vi "Main.vi"(8 "error in":errorcluster, 11 "gRPC Client in":refnum<class "gRPC Client.lvclass">) -> (0 "error out":errorcluster, 3 "gRPC Client out":refnum<class "gRPC Client.lvclass">)   [LabVIEW 2023, in "gRPC Client.lvclass"]
doc: "The <b>Queued Message Handler</b> of the Worker that owns this VI."
uses:
  gRPC Client.lvclass
  C:/Program Files (x86)/National Instruments/LabVIEW 2023/vi.lib/addons/_Workers/Library/Classes/Worker/Worker.lvclass
  Generated_client/RPC Messages/streamai_signalConfig.ctl
  Generated_client/RPC Messages/streamai_SignalType.ctl
  Generated_client/RPC Messages/streamai_samplingConfig.ctl
  Initialization Data.ctl
  Response Cases.ctl
  <vilib>/gRPC/LabVIEW gRPC Library/Shared/grpcId.ctl
  gRPC Client.lvclass/gRPC Client.ctl
  <vilib>/addons/_Workers/Library/Classes/Message Queue/Message Queue.lvclass
  Generated_client/Generated_client.lvlib
  <vilib>/gRPC/LabVIEW gRPC Library/grpc-lvsupport-release.lvlib
panel:
  in  "Start Acq":bool
  in  "Address":string="localhost:50051"
  in  "Start Button":bool
  in  "Sampling Config":T1={"sample_rate"=100.0, "num_sample"=100}
  in  "Signal Config":T2={"type"=enum."SIGNAL_SQUARE", "offset"=0.0, "frequency"=5.0, "amplitude"=2.0}
  out "Waveform Chart":waveform(dbl)(graph)
  # "gRPC Client"
  # "Connector Pane"
  # "Locals"
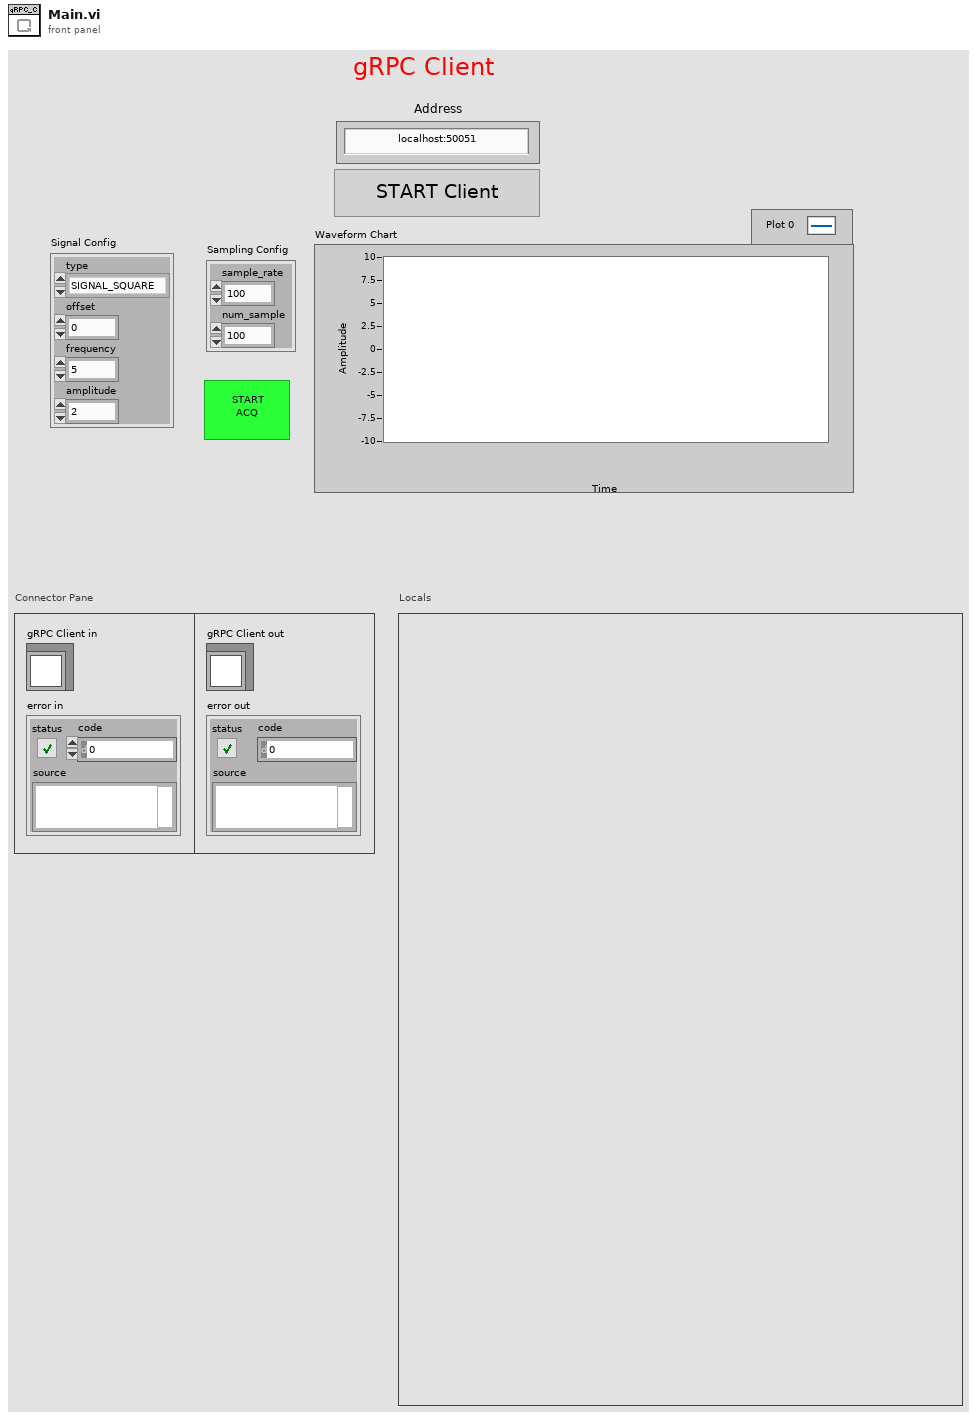
[diagram p1: front panel]
types:
  T1 = typedef "Generated_client.lvlib/streamai_samplingConfig.ctl" = cluster{"sample_rate":dbl, "num_sample":i32}
  T2 = typedef "Generated_client.lvlib/streamai_signalConfig.ctl" = cluster{"type":T3, "offset":dbl, "frequency":dbl, "amplitude":dbl}
  T3 = typedef "Generated_client.lvlib/streamai_SignalType.ctl" = enum32{"SIGNAL_SINE", "SIGNAL_SQUARE"}
  T4 = enum32{"Invalid", "Standard", "Closed", "Hidden", "Minimized", "Maximized"}
  T5 = typedef "gRPC Client.lvclass/Initialization Data.ctl" = cluster{"Response Cases":T6}
  T6 = typedef "gRPC Client.lvclass/Response Cases.ctl" = cluster{"gRPC ID":T7, "Call Id":T7}
  T7 = typedef "grpc-lvsupport-release.lvlib/grpcId.ctl" = u64
  T8 = enum8{"Enabled", "Disabled", "Disabled and Grayed Out"}
  T9 = typedef "Generated_client.lvlib/streamai_waveform.ctl" = cluster{"t0":T10, "delta_t":dbl, "values":dbl[]}
  T10 = typedef "Generated_client.lvlib/google_protobuf_Timestamp.ctl" = cluster{"seconds":i64, "nanos":i32}
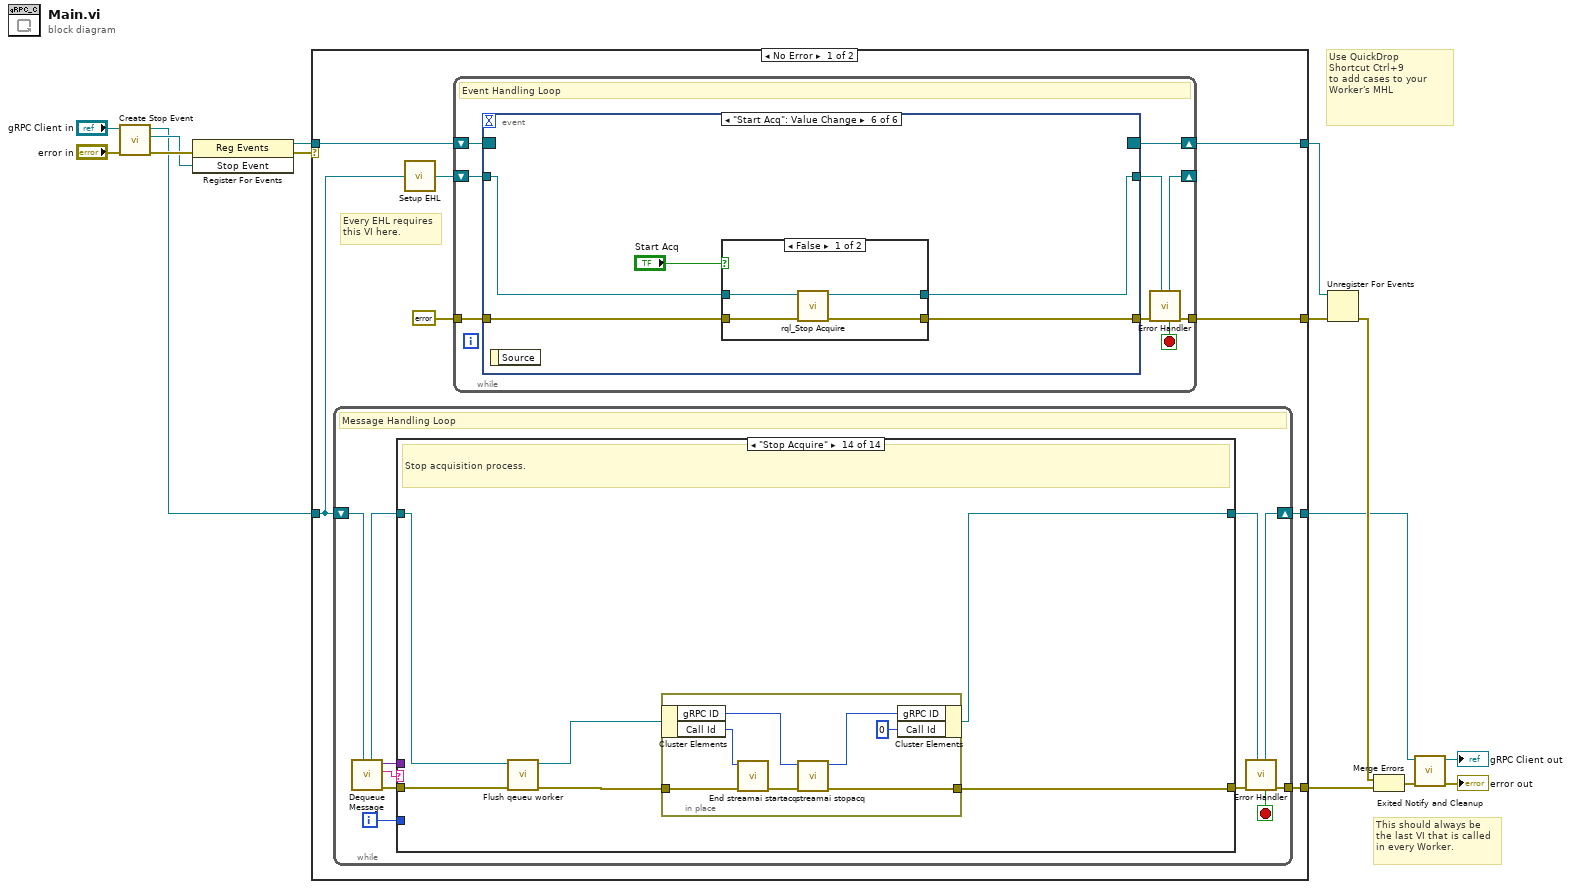
[diagram p0: block diagram]
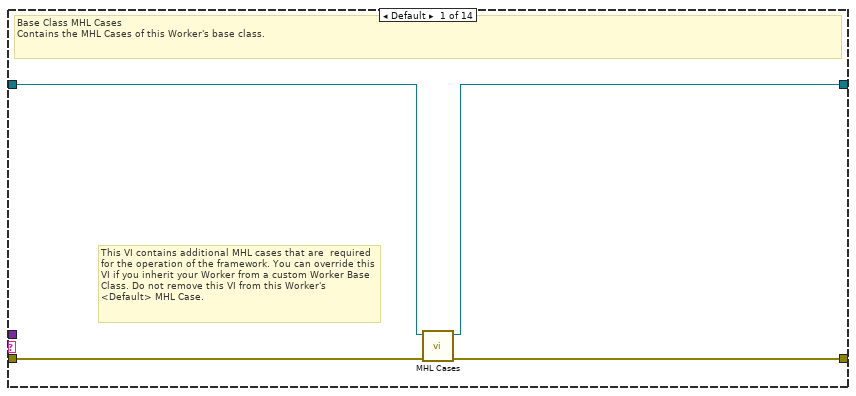
[diagram p2: hidden frame]
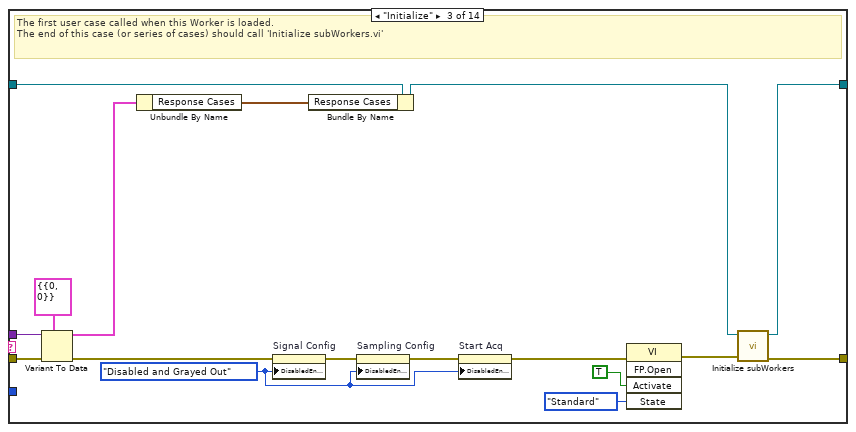
[diagram p4: hidden frame]
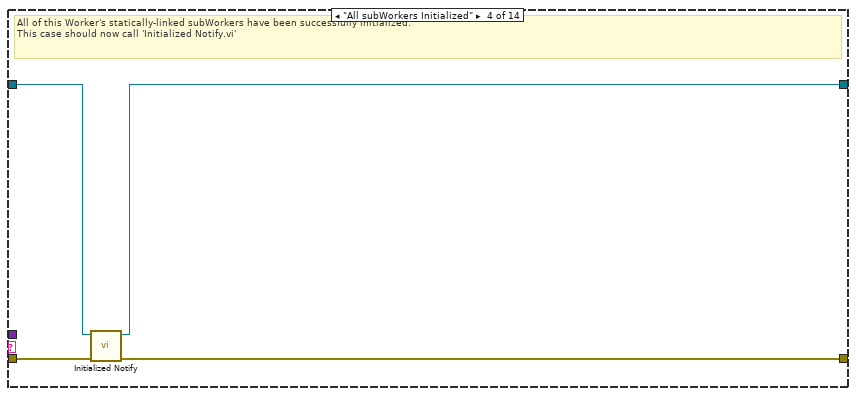
[diagram p5: hidden frame]
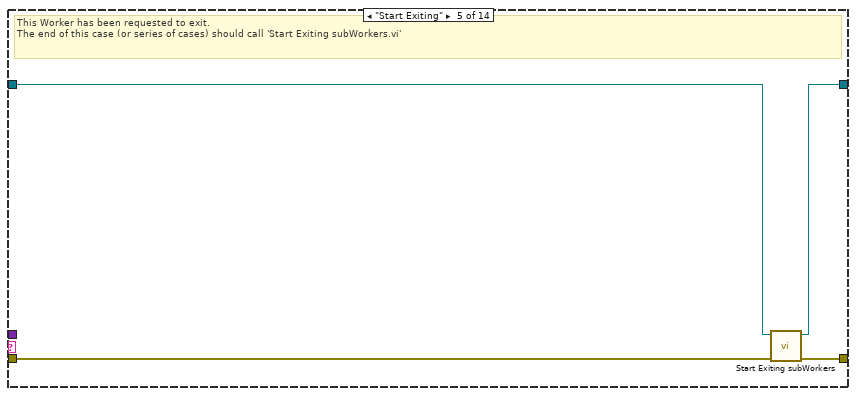
[diagram p6: hidden frame]
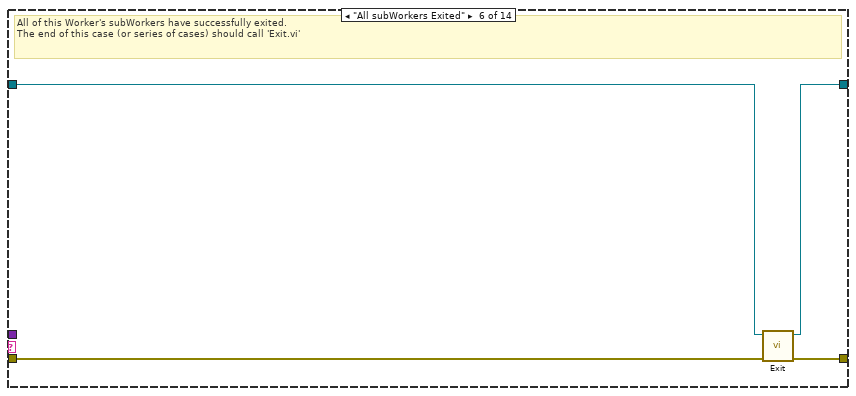
[diagram p7: hidden frame]
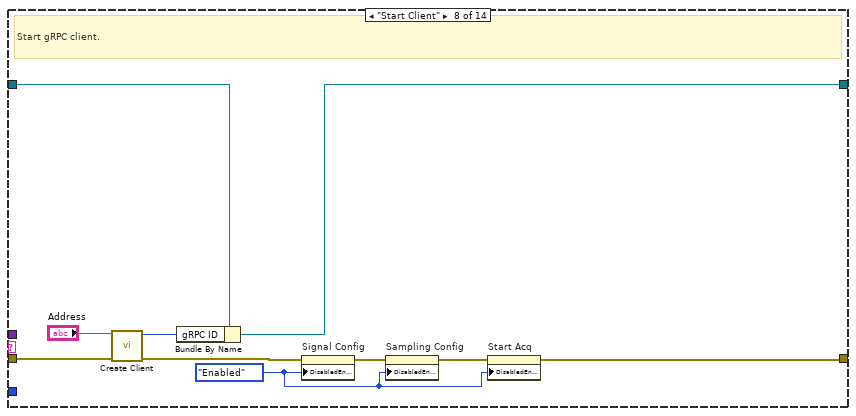
[diagram p9: hidden frame]
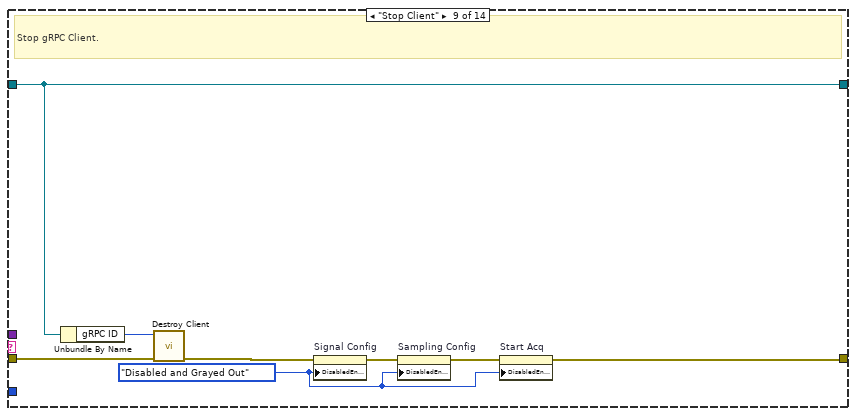
[diagram p10: hidden frame]
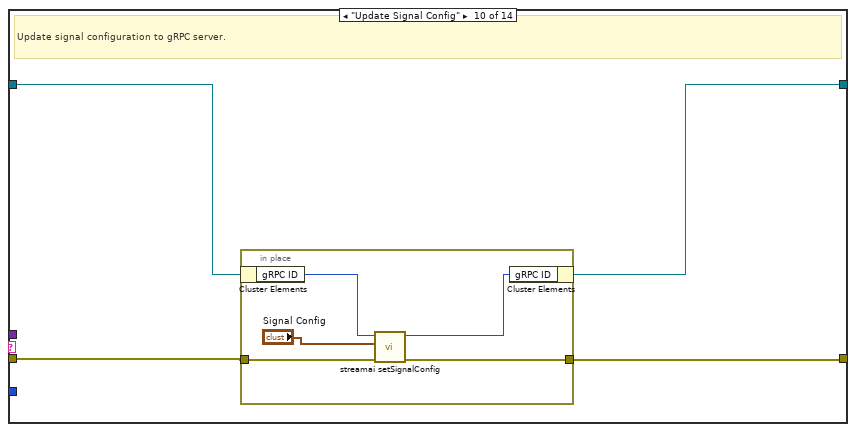
[diagram p11: hidden frame]
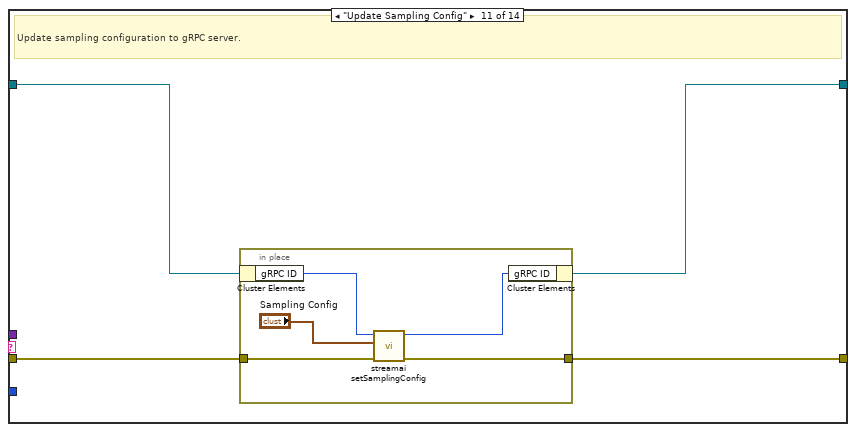
[diagram p12: hidden frame]
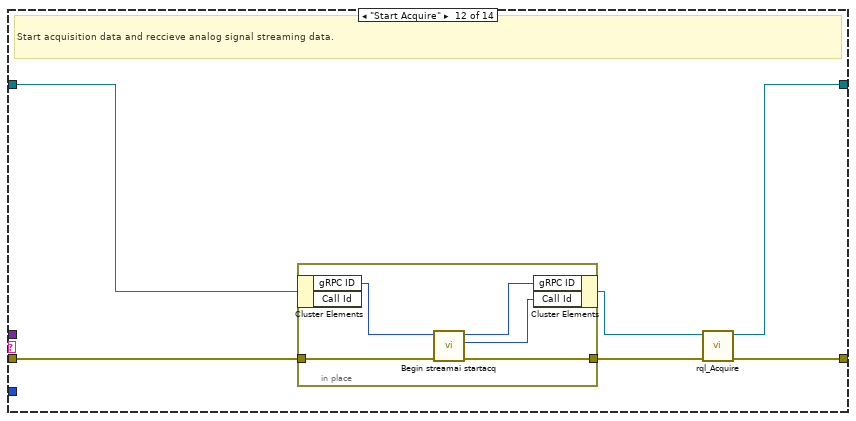
[diagram p13: hidden frame]
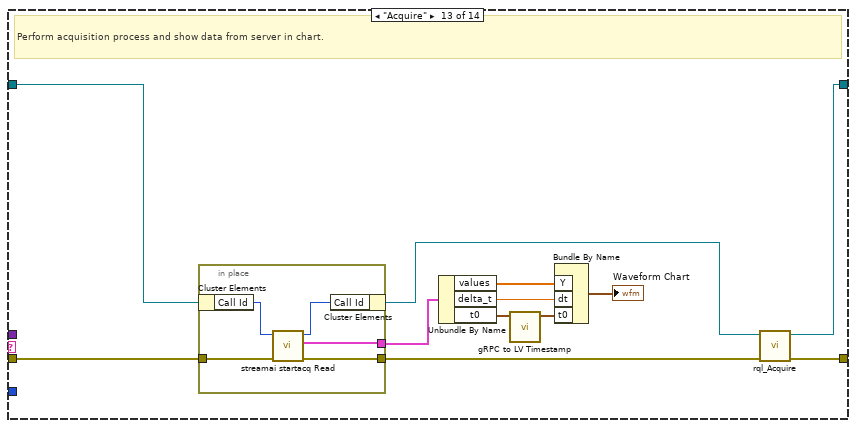
[diagram p14: hidden frame]
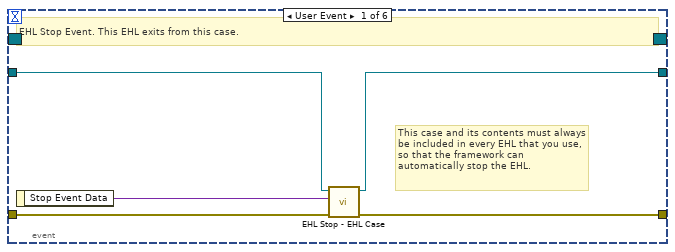
[diagram p15: hidden frame]
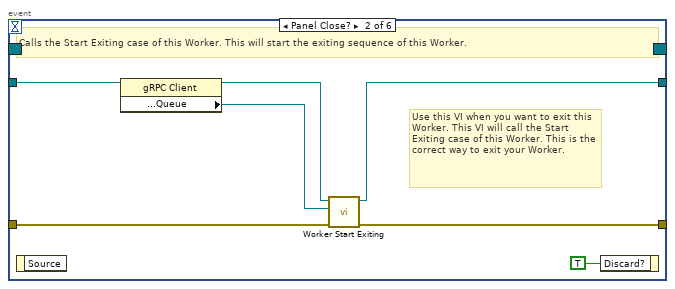
[diagram p16: hidden frame]
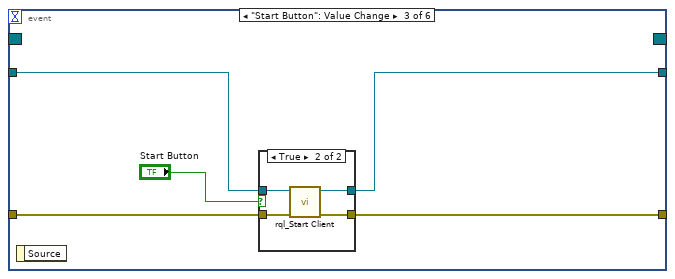
[diagram p17: hidden frame]
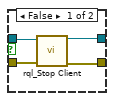
[diagram p18: hidden frame]
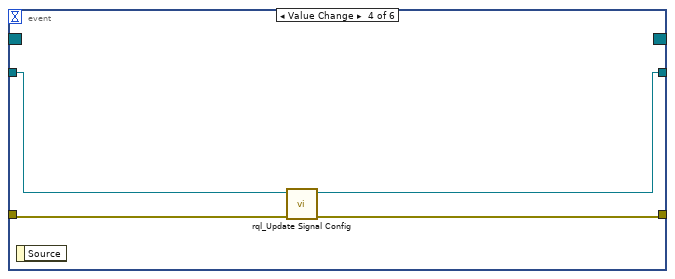
[diagram p19: hidden frame]
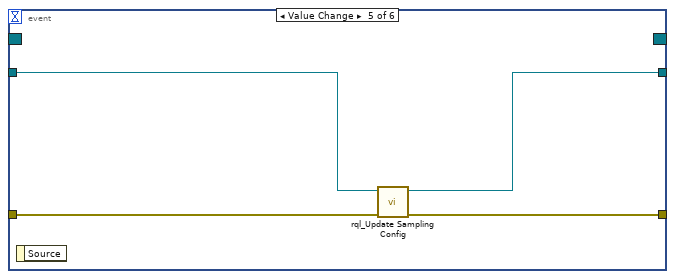
[diagram p20: hidden frame]
diagram:
  # "Use QuickDrop\nShortcut Ctrl+9\nto add cases to your\nWorker's MHL"
  # "This should always be the last VI that is called in every Worker."
  n1 = call-dynamic "Create Stop Event.vi"("error in"="error in", "Worker"="gRPC Client in") -> ("error out"=w10:errorcluster, "Stop Event"=w7:refnum<user-event>, "Worker out"=w4:refnum<class "gRPC Client.lvclass">)  [unwired: 7 in]
  n2 = register-events(error in=w10, w7) -> (reference out=w9:refnum<event-registration>, error out=w1:errorcluster)  [unwired: 1 in]
  n3 = case shown="No Error" w1 {
    tunnel: w4 -> [w18 w205]
    tunnel: [w16 w206] -> w8
    tunnel: w9 -> [w23 w207]
    tunnel: [w20 w208] -> w14
    tunnel: [w22 w207] -> w13
    tunnel: [w17 w204] -> w11
    selector: w1 -> [_ w208]
    frame No Error {
      # "Every EHL requires\nthis VI here."
      n4 = while {
        shift-right: [w32] -> w17
        shift-left: w18 -> [w34]
        tunnel: [w33] -> w16
        i -> [w25]
        stop <- w26 stop-if-true
        # "Message Handling Loop"
        n5 = call-dynamic "Dequeue Message.vi"("Worker"=w34) -> ("error out"=w31:errorcluster, "Case out"=w27:string, "Data out"=w24:variant, "Worker out"=w29:refnum<class "gRPC Client.lvclass">)  [unwired: 6 in, 1 out]
        n6 = case "Worker MHL Case Structure (DO NOT CHANGE LABEL NAME)" shown="\"Stop Acquire\"" w27 {
          tunnel: w31 -> [w38 w39 w55 w59 w62 w69 w71 w77 w86 w93 w102 w113 w130 w137]
          tunnel: [w37 w39 w57 w58 w65 w68 w71 w74 w84 w92 w101 w110 w121 w141] -> w30
          tunnel: w29 -> [w36 w40 w54 w61 w63 w67 w70 w81 w83 w91 w100 w111 w128 w139]
          tunnel: [w35 w40 w56 w60 w64 w66 w70 w73 w83 w90 w99 w108 w119 w140] -> w28
          tunnel: w25 -> [_ _ _ _ _ _ _ _ _ _ _ _ _ _]
          tunnel: w24 -> [_ _ w53 _ _ _ _ _ _ _ _ _ _ _]
          frame Default {
            # "This VI contains additional MHL cases that are  required for the operation of the framework. You can override this VI if you inherit your Worker from a custom Worker Base Class. Do not remove this VI from this Worker's <Default> MHL Case."
            # "Base Class MHL Cases\nContains the MHL Cases of this Worker's base class."
            n7 = call-dynamic "MHL Cases.vi"("error in"=w38, "Worker in"=w36) -> ("error out"=w37:errorcluster, "Worker out"=w35:refnum<class "gRPC Client.lvclass">)  [unwired: 8 in]
          }
          frame "------------ FRAMEWORK CASES -----------" {
            # "Start of Workers Framework Cases"
          }
          frame "Initialize" {
            w45 = T8."Disabled and Grayed Out" ("Disabled")
            # "The first user case called when this Worker is loaded.\nThe end of this case (or series of cases) should call 'Initialize subWorkers.vi'"
            n8 = Variant To Data(error in=w55, type=T5 {"Response Cases"={"gRPC ID"=0, "Call Id"=0}} ("Initialization Data"), Variant=w53) -> (data=w51:T5, error out=w46:errorcluster)
            n9 = Unbundle By Name(w51) -> ("Response Cases"=w50:T6)
            n10 = property on="Signal Config" class="Clust (strict)"(error in=w46, "DisabledEnum"=w45) -> (error out=w48:errorcluster)  [unwired: 1 in, 1 out]
            n11 = Bundle By Name(cluster=w54, "Response Cases"=w50) -> (w52:refnum<class "gRPC Client.lvclass">)
            n12 = property on="Sampling Config" class="Clust (strict)"(error in=w48, "DisabledEnum"=w45) -> (error out=w47:errorcluster)  [unwired: 1 in, 1 out]
            n13 = property on="Start Acq" class="Bool (strict)"(error in=w47, "DisabledEnum"=w45) -> (error out=w42:errorcluster)  [unwired: 1 in, 1 out]
            n14 = invoke class="VI" method="FP.Open"(error in=w42, "Activate"=TRUE ("Activate?"), "State"=T4."Standard") -> (error out=w41:errorcluster)  [unwired: 2 in, 4 out]
            n15 = call-dynamic "Initialize subWorkers.vi"("error in"=w41, "Worker"=w52) -> ("error out"=w57:errorcluster, "dup Worker out"=w56:refnum<class "gRPC Client.lvclass">)  [unwired: 8 in]
          }
          frame "All subWorkers Initialized" {
            # "All of this Worker's statically-linked subWorkers have been successfully initialized.\nThis case should now call 'Initialized Notify.vi'"
            n16 = call-dynamic "Initialized Notify.vi"("error in"=w59, "Worker"=w61) -> ("error out"=w58:errorcluster, "dup Worker out"=w60:refnum<class "gRPC Client.lvclass">)  [unwired: 8 in]
          }
          frame "Start Exiting" {
            # "This Worker has been requested to exit. \nThe end of this case (or series of cases) should call 'Start Exiting subWorkers.vi'"
            n17 = call-dynamic "Start Exiting subWorkers.vi"("error_in"=w62, "Worker"=w63) -> ("error out"=w65:errorcluster, "dup Worker out"=w64:refnum<class "gRPC Client.lvclass">)  [unwired: 8 in]
          }
          frame "All subWorkers Exited" {
            # "All of this Worker's subWorkers have successfully exited. \nThe end of this case (or series of cases) should call 'Exit.vi'"
            n18 = call-dynamic "Exit.vi"("error_in"=w69, "Worker"=w67) -> ("error out"=w68:errorcluster, "dup Worker out"=w66:refnum<class "gRPC Client.lvclass">)  [unwired: 8 in]
          }
          frame "------------- LOCAL API CASES -------------" {
            # "Start of Workers Local API Cases"
          }
          frame "Start Client" {
            w78 = T8."Enabled" ("Disabled")
            # "Start gRPC client."
            n19 = call "Create Client.vi"("error in"=w77, "address"="Address") -> ("error out"=w76:errorcluster, "gRPC ID Out"=w72:T7)  [unwired: 8 in]
            n20 = Bundle By Name(cluster=w81, "gRPC ID"=w72) -> (w73:refnum<class "gRPC Client.lvclass">)
            n21 = property on="Signal Config" class="Clust (strict)"(error in=w76, "DisabledEnum"=w78) -> (error out=w80:errorcluster)  [unwired: 1 in, 1 out]
            n22 = property on="Sampling Config" class="Clust (strict)"(error in=w80, "DisabledEnum"=w78) -> (error out=w79:errorcluster)  [unwired: 1 in, 1 out]
            n23 = property on="Start Acq" class="Bool (strict)"(error in=w79, "DisabledEnum"=w78) -> (error out=w74:errorcluster)  [unwired: 1 in, 1 out]
          }
          frame "Stop Client" {
            w87 = T8."Disabled and Grayed Out" ("Disabled")
            # "Stop gRPC Client."
            n24 = Unbundle By Name(w83) -> ("gRPC ID"=w82:T7)
            n25 = call "Destroy Client.vi"("error in"=w86, "gRPC ID"=w82) -> ("error out"=w85:errorcluster)  [unwired: 9 in]
            n26 = property on="Signal Config" class="Clust (strict)"(error in=w85, "DisabledEnum"=w87) -> (error out=w89:errorcluster)  [unwired: 1 in, 1 out]
            n27 = property on="Sampling Config" class="Clust (strict)"(error in=w89, "DisabledEnum"=w87) -> (error out=w88:errorcluster)  [unwired: 1 in, 1 out]
            n28 = property on="Start Acq" class="Bool (strict)"(error in=w88, "DisabledEnum"=w87) -> (error out=w84:errorcluster)  [unwired: 1 in, 1 out]
          }
          frame "Update Signal Config" {
            # "Update signal configuration to gRPC server."
            n29 = in-place {
              in-place-border: w93 -> [w98]
              in-place-border: [w97] -> w92
              n30 = in-place-cluster #1(w91) -> ("gRPC ID"=w96:T7)
              n31 = call "streamai setSignalConfig.vi"("error in"=w98, "Request Data"="Signal Config", "gRPC ID"=w96) -> ("error out"=w97:errorcluster, "gRPC ID out"=w95:T7)  [unwired: 6 in, 1 out]
              n32 = in-place-cluster #1("gRPC ID"=w95) -> (w90:refnum<class "gRPC Client.lvclass">)
            }
          }
          frame "Update Sampling Config" {
            # "Update sampling configuration to gRPC server."
            n33 = in-place {
              in-place-border: w102 -> [w107]
              in-place-border: [w106] -> w101
              n34 = in-place-cluster #2(w100) -> ("gRPC ID"=w105:T7)
              n35 = call "streamai setSamplingConfig.vi"("error in"=w107, "Request Data"="Sampling Config", "gRPC ID"=w105) -> ("error out"=w106:errorcluster, "gRPC ID out"=w104:T7)  [unwired: 6 in, 1 out]
              n36 = in-place-cluster #2("gRPC ID"=w104) -> (w99:refnum<class "gRPC Client.lvclass">)
            }
          }
          frame "Start Acquire" {
            # "Start acquisition data and reccieve analog signal streaming data."
            n37 = in-place {
              in-place-border: w113 -> [w118]
              in-place-border: [w117] -> w112
              n38 = in-place-cluster #3(w111) -> ("gRPC ID"=w115:T7)  [unwired: 1 out]
              n39 = call "Begin streamai startacq.vi"("error in"=w118, "gRPC ID"=w115) -> ("error out"=w117:errorcluster, "Call Id Out"=w114:T7, "gRPC ID out"=w116:T7)  [unwired: 7 in]
              n40 = in-place-cluster #3("gRPC ID"=w116, "Call Id"=w114) -> (w109:refnum<class "gRPC Client.lvclass">)
            }
            n41 = call "rql_Acquire.vi"("error in"=w112, "gRPC Client in"=w109) -> ("error out"=w110:errorcluster, "dup gRPC Client out"=w108:refnum<class "gRPC Client.lvclass">)  [unwired: 8 in]
          }
          frame "Acquire" {
            # "Perform acquisition process and show data from server in chart."
            n42 = in-place {
              in-place-border: w130 -> [w135]
              in-place-border: [w134] -> w129
              in-place-border: [w131] -> w127
              n43 = in-place-cluster #4(w128) -> ("Call Id"=w133:T7)
              n44 = call "streamai startacq Read.vi"("error in"=w135, "Call ID in"=w133) -> ("error out"=w134:errorcluster, "Response Data"=w131:T9, "Call ID"=w132:T7)  [unwired: 6 in, 1 out]
              n45 = in-place-cluster #4("Call Id"=w132) -> (w120:refnum<class "gRPC Client.lvclass">)
            }
            n46 = Unbundle By Name(w127) -> ("values"=w126:dbl[], "delta_t"=w125:dbl, "t0"=w124:T10)
            n47 = call "gRPC to LV Timestamp.vi"("gRPC Timestamp"=w124) -> ("LV Timestamp"=w123:timestamp)  [unwired: 10 in]
            n48 = Bundle By Name("Y"=w126, "dt"=w125, "t0"=w123) -> (→"Waveform Chart":waveform(dbl))  [unwired: 1 in]
            n49 = call "rql_Acquire.vi"("error in"=w129, "gRPC Client in"=w120) -> ("error out"=w121:errorcluster, "dup gRPC Client out"=w119:refnum<class "gRPC Client.lvclass">)  [unwired: 8 in]
          }
          frame "Stop Acquire" {
            # "Stop acquisition process."
            n50 = call "Flush qeueu worker.vi"("error in (no error)"=w137, "gRPC Client in"=w139) -> ("error out"=w136:errorcluster, "reference out"=w138:refnum<class "gRPC Client.lvclass">)  [unwired: 8 in]
            n51 = in-place {
              in-place-border: w136 -> [w148]
              in-place-border: [w147] -> w141
              n52 = in-place-cluster #5(w138) -> ("gRPC ID"=w145:T7, "Call Id"=w143:T7)
              n53 = call "End streamai startacq.vi"("error in"=w148, "Call ID in"=w143) -> ("error out"=w144:errorcluster)  [unwired: 8 in, 1 out]
              n54 = call "streamai stopacq.vi"("error in"=w144, "gRPC ID"=w145) -> ("error out"=w147:errorcluster, "gRPC ID out"=w146:T7)  [unwired: 7 in, 1 out]
              n55 = in-place-cluster #5("gRPC ID"=w146, "Call Id"=T7 0 ("Response Cases.Call Id")) -> (w140:refnum<class "gRPC Client.lvclass">)
            }
          }
        }
        n56 = call-dynamic "Error Handler.vi"("Worker"=w28, "error_in"=w30) -> ("error out"=w33:errorcluster, "Stop Loop"=w26:bool, "Worker out"=w32:refnum<class "gRPC Client.lvclass">)  [unwired: 7 in]
      }
      n57 = call-dynamic "Setup EHL.vi"("Worker"=w18) -> ("Worker out"=w19:refnum<class "gRPC Client.lvclass">)  [unwired: 14 in]
      n58 = while "Event Handling Loop" {
        shift-right: [w157] -> w22
        shift-left: w23 -> [w156]
        tunnel: [w152] -> w20
        tunnel: errorcluster {"status"=FALSE, "code"=0, "source"=""} ("error constant") -> [w154]
        shift-right: [w150] -> _
        shift-left: w19 -> [w155]
        stop <- w149 stop-if-true
        # "Event Handling Loop"
        n59 = event shown="[5] \"Start Acq\": Value Change" {
          selector: w156 -> [_ _ _ _ _ _]
          dyn-events: [_ _ _ _ _ _] -> w157
          timeout: _ -> [_ _ _ _ _ _]
          tunnel: [w161 w168 w173 w185 w189 w194] -> w153
          tunnel: w154 -> [w162 w167 w174 w186 w190 w195]
          tunnel: w155 -> [w160 w166 w172 w184 w187 w193]
          tunnel: [w159 w165 w171 w183 w188 w192] -> w151
          event User Event {
            # "This case and its contents must always be included in every EHL that you use, so that the framework can automatically stop the EHL."
            # "EHL Stop Event. This EHL exits from this case."
            n60 = event-data() -> ("Stop Event Data"=w158:variant)  [unwired: 1 in]
            n61 = call-dynamic "EHL Stop - EHL Case.vi"("error in"=w162, "Stop Event Data"=w158, "Worker"=w160) -> ("error out"=w161:errorcluster, "Worker out"=w159:refnum<class "gRPC Client.lvclass">)  [unwired: 7 in]
          }
          event Panel Close? {
            # "Use this VI when you want to exit this Worker. This VI will call the Start Exiting case of this Worker. This is the correct way to exit your Worker."
            # "Calls the Start Exiting case of this Worker. This will start the exiting sequence of this Worker."
            n62 = event-data() -> ()  [unwired: 1 in, 1 out]
            n63 = property class="gRPC Client"(reference=w166) -> (reference out=w164:refnum<class "gRPC Client.lvclass">, "Accessors:Read:Public API:Queue"=w163:refnum<class "Message Queue.lvclass">)  [unwired: 1 in, 1 out]
            n64 = call-dynamic "Worker Start Exiting.vi"("error_in"=w167, "Message Queue"=w163, "Worker"=w164) -> ("error out"=w168:errorcluster, "dup Worker out"=w165:refnum<class "gRPC Client.lvclass">)  [unwired: 7 in]
            n65 = event-data("Discard?"=TRUE) -> ()  [unwired: 1 in, 1 out]
          }
          event "Start Button": Value Change {
            n66 = event-data() -> ()  [unwired: 1 in, 1 out]
            n67 = case shown="True" "Start Button" {
              tunnel: w174 -> [w178 w182]
              tunnel: [w177 w181] -> w173
              tunnel: w172 -> [w175 w180]
              tunnel: [w176 w179] -> w171
              frame False {
                n68 = call "rql_Stop Client.vi"("error in"=w178, "gRPC Client in"=w175) -> ("error out"=w177:errorcluster, "dup gRPC Client out"=w176:refnum<class "gRPC Client.lvclass">)  [unwired: 8 in]
              }
              frame True {
                n69 = call "rql_Start Client.vi"("error in"=w182, "gRPC Client in"=w180) -> ("error out"=w181:errorcluster, "dup gRPC Client out"=w179:refnum<class "gRPC Client.lvclass">)  [unwired: 8 in]
              }
            }
          }
          event Value Change {
            n70 = event-data() -> ()  [unwired: 1 in, 1 out]
            n71 = call "rql_Update Signal Config.vi"("error in"=w186, "gRPC Client in"=w184) -> ("error out"=w185:errorcluster, "dup gRPC Client out"=w183:refnum<class "gRPC Client.lvclass">)  [unwired: 8 in]
          }
          event Value Change {
            n72 = event-data() -> ()  [unwired: 1 in, 1 out]
            n73 = call "rql_Update Sampling Config.vi"("error in"=w190, "gRPC Client in"=w187) -> ("error out"=w189:errorcluster, "dup gRPC Client out"=w188:refnum<class "gRPC Client.lvclass">)  [unwired: 8 in]
          }
          event "Start Acq": Value Change {
            n74 = event-data() -> ()  [unwired: 1 in, 1 out]
            n75 = case shown="False" "Start Acq" {
              tunnel: w195 -> [w199 w203]
              tunnel: [w198 w202] -> w194
              tunnel: w193 -> [w196 w201]
              tunnel: [w197 w200] -> w192
              frame False {
                n76 = call "rql_Stop Acquire.vi"("error in"=w199, "gRPC Client in"=w196) -> ("error out"=w198:errorcluster, "dup gRPC Client out"=w197:refnum<class "gRPC Client.lvclass">)  [unwired: 8 in]
              }
              frame True {
                n77 = call "rql_Start Acquire.vi"("error in"=w203, "gRPC Client in"=w201) -> ("error out"=w202:errorcluster, "dup gRPC Client out"=w200:refnum<class "gRPC Client.lvclass">)  [unwired: 8 in]
              }
            }
          }
        }
        n78 = call-dynamic "Error Handler.vi"("Worker"=w151, "error_in"=w153) -> ("error out"=w152:errorcluster, "Stop Loop"=w149:bool, "Worker out"=w150:refnum<class "gRPC Client.lvclass">)  [unwired: 7 in]
      }
    }
    frame Error {
      n79 = call-dynamic "Error Handler.vi"("Worker"=w205, "error_in"=w208) -> ("error out"=w206:errorcluster, "Worker out"=w204:refnum<class "gRPC Client.lvclass">)  [unwired: 7 in, 1 out]
    }
  }
  n80 = Unregister For Events(event registration refnum=w13, error in=w14) -> (error out=w15:errorcluster)
  n81 = Merge Errors(w15, w8) -> (w12:errorcluster)
  n82 = call-dynamic "Exited Notify and Cleanup.vi"("error_in"=w12, "Worker"=w11) -> ("error out"=→"error out":errorcluster, "dup Worker out"=→"gRPC Client out":refnum<class "gRPC Client.lvclass">)  [unwired: 8 in]
